vi "ODX_Ablaufbefehl.vi"(9 "Operand in":u32, 10 "Carry in":bool, 11 "SA2 Operator":T1[](array[typedef]) {"Wert" format="%.0x"}) -> (1 "Operand out":u32, 2 "Carry out":bool, 3 "SA2 Operator out":T1[](array[typedef]) {"Wert" format="%.0x"})   [LabVIEW 2014]
uses:
  Typedefs/Diagnose_SA2_Rechnenbefehl.ctl
  Typedefs/Diagnose_SA2_Operation_ENUM.ctl
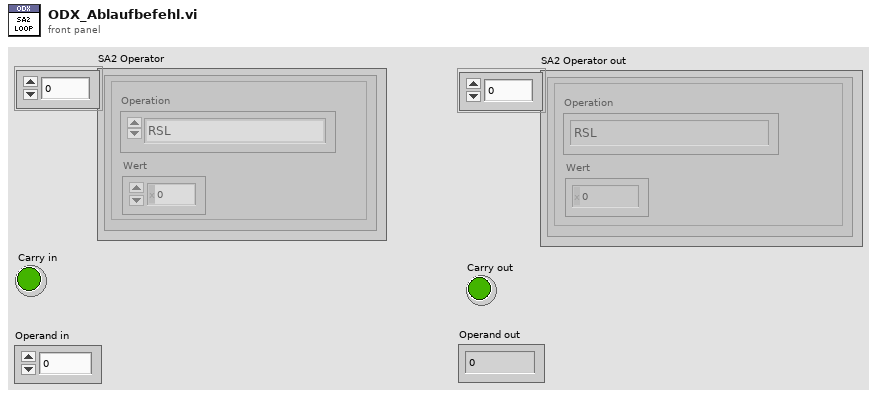
[diagram p1: front panel]
types:
  T1 = typedef "Diagnose_SA2_Rechnenbefehl.ctl" = cluster{"Operation":T2, "Wert":u32}
  T2 = typedef "Diagnose_SA2_Operation_ENUM.ctl" = enum16{"RSL", "RSR", "ADD", "SUB", "EOR", "Durchläufe", "NEXT", "BCC", "BRA", "Fertig"}
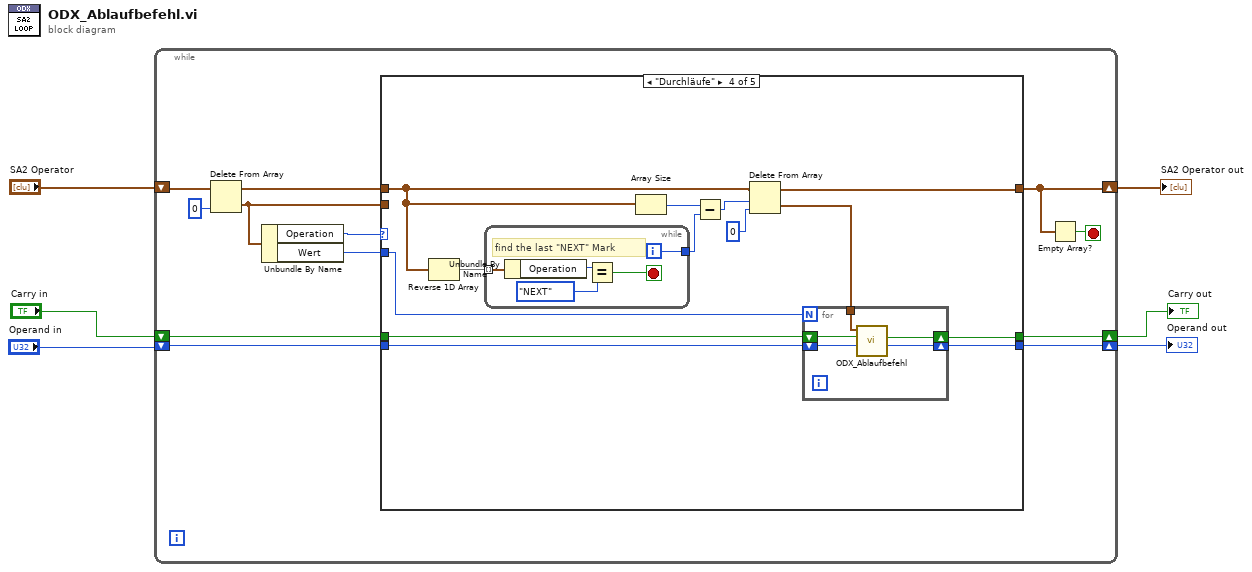
[diagram p0: block diagram]
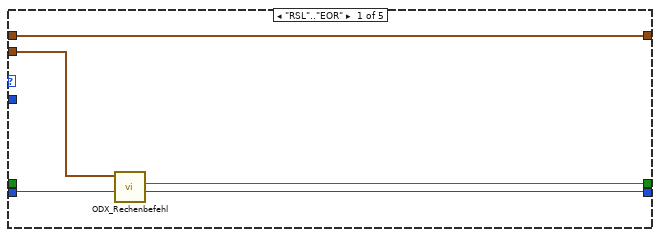
[diagram p2: hidden frame]
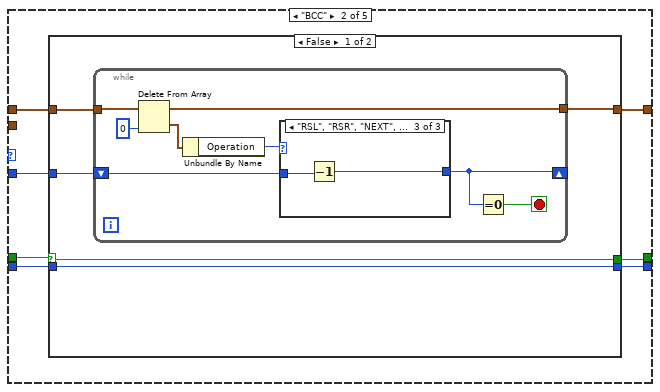
[diagram p3: hidden frame]
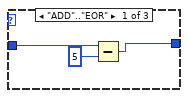
[diagram p4: hidden frame]
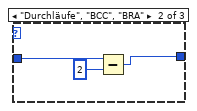
[diagram p5: hidden frame]
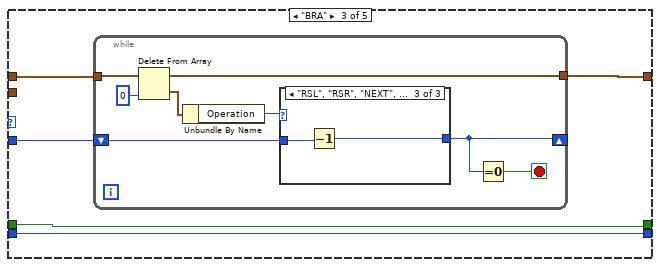
[diagram p7: hidden frame]
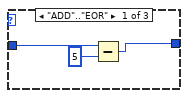
[diagram p8: hidden frame]
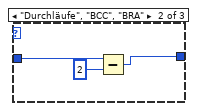
[diagram p9: hidden frame]
diagram:
  n1 = while {
    shift-right: [w16] -> w6
    shift-left: "Operand in" -> [w15]
    shift-right: [w7] -> w3
    shift-left: "SA2 Operator" -> [w14]
    shift-right: [w10] -> w1
    shift-left: "Carry in" -> [w9]
    stop <- w8 stop-if-true
    n2 = Delete From Array(array=w14, index=0) -> (deleted portion=w12:T1, array with subset deleted=w11:T1[])  [unwired: 1 in]
    n3 = Unbundle By Name(w12) -> ("Operation"=w18:T2, "Wert"=w17:u32)
    n4 = case shown="\"Durchläufe\"" w18 {
      tunnel: w17 -> [_ w24 w55 w76 _]
      tunnel: [w22 w28 w59 w79 w99] -> w16
      tunnel: w15 -> [w23 w29 w59 w80 w99]
      tunnel: w12 -> [w21 _ _ _ _]
      tunnel: w11 -> [w20 w27 w58 w85 w101]
      tunnel: [w20 w26 w57 w82 w101] -> w7
      tunnel: [w19 w25 w56 w78 w100] -> w10
      tunnel: w9 -> [_ w30 w56 w77 w100]
      frame "RSL".."EOR" {
        n5 = call "ODX_Rechenbefehl.vi"("Operand in"=w23, "operation"=w21) -> ("Operand out"=w22:u32, "Carry"=w19:bool)  [unwired: 8 in]
      }
      frame "BCC" {
        n6 = case shown="False" w30 {
          selector: w30 -> [w34 w52]
          tunnel: w29 -> [w35 w54]
          tunnel: [w35 w54] -> w28
          tunnel: [w31 w53] -> w26
          tunnel: w27 -> [w32 w53]
          tunnel: [w34 w52] -> w25
          tunnel: w24 -> [w33 _]
          frame False {
            n7 = while {
              shift-right: [w37] -> _
              shift-left: w33 -> [w38]
              tunnel: w32 -> [w43]
              tunnel: [w41] -> w31
              stop <- w36 stop-if-true
              n8 = Delete From Array(array=w43, index=0) -> (deleted portion=w40:T1, array with subset deleted=w41:T1[])  [unwired: 1 in]
              n9 = Unbundle By Name(w40) -> ("Operation"=w39:T2)
              n10 = case shown="\"RSL\", \"RSR\", \"NEXT\", \"Fertig\"" w39 {
                tunnel: w38 -> [w46 w49 w51]
                tunnel: [w44 w47 w50] -> w37
                frame "ADD".."EOR" {
                  n11 = Subtract(x=w46, y=u32 5) -> (x-y=w44:u32)
                }
                frame "Durchläufe", "BCC", "BRA" {
                  n12 = Subtract(x=w49, y=u32 2) -> (x-y=w47:u32)
                }
                frame "RSL", "RSR", "NEXT", "Fertig" {
                  n13 = Decrement(x=w51) -> (x-1=w50:u32)
                }
              }
              n14 = Equal To 0?(x=w37) -> (x = 0?=w36:bool)
            }
          }
          frame True {
          }
        }
      }
      frame "BRA" {
        n15 = while {
          shift-right: [w61] -> _
          shift-left: w55 -> [w62]
          tunnel: w58 -> [w67]
          tunnel: [w65] -> w57
          stop <- w60 stop-if-true
          n16 = Delete From Array(array=w67, index=0) -> (deleted portion=w64:T1, array with subset deleted=w65:T1[])  [unwired: 1 in]
          n17 = Unbundle By Name(w64) -> ("Operation"=w63:T2)
          n18 = case shown="\"RSL\", \"RSR\", \"NEXT\", \"Fertig\"" w63 {
            tunnel: w62 -> [w70 w73 w75]
            tunnel: [w68 w71 w74] -> w61
            frame "ADD".."EOR" {
              n19 = Subtract(x=w70, y=u32 5) -> (x-y=w68:u32)
            }
            frame "Durchläufe", "BCC", "BRA" {
              n20 = Subtract(x=w73, y=u32 2) -> (x-y=w71:u32)
            }
            frame "RSL", "RSR", "NEXT", "Fertig" {
              n21 = Decrement(x=w75) -> (x-1=w74:u32)
            }
          }
          n22 = Equal To 0?(x=w61) -> (x = 0?=w60:bool)
        }
      }
      frame "Durchläufe" {
        n23 = Reverse 1D Array(array=w85) -> (reversed array=w88:T1[])
        n24 = while {
          tunnel: w88 -> [w98] mode=indexing
          tunnel: [w94] -> w86
          i -> [w94]
          stop <- w95 stop-if-true
          # "find the last \"NEXT\" Mark"
          n25 = Unbundle By Name(w98) -> ("Operation"=w97:T2)
          n26 = Equal?(x=w97, y=Diagnose_SA2_Operation_ENUM."NEXT") -> (x = y?=w95:bool)
        }
        n27 = Array Size(array=w85) -> (size(s)=w87:i32)
        n28 = Subtract(x=w87, y=w86) -> (x-y=w84:i32)
        n29 = Delete From Array(array=w85, length=w84, index=0) -> (deleted portion=w81:T1[], array with subset deleted=w82:T1[])
        n30 = for {
          N: w76 -> [_]
          tunnel: w81 -> [w93]
          shift-right: [w91] -> w79
          shift-left: w80 -> [w92]
          shift-right: [w90] -> w78
          shift-left: w77 -> [w89]
          n31 = call "ODX_Ablaufbefehl.vi"("Operand in"=w92, "Carry in"=w89, "SA2 Operator"=w93) -> ("Operand out"=w91:u32, "Carry out"=w90:bool)  [unwired: 6 in, 1 out]
        }
      }
      frame "NEXT", "Fertig" {
      }
    }
    n32 = Empty Array?(array=w7) -> (empty?=w8:bool)
  }
  "Operand out" <- w6
  "SA2 Operator out" <- w3
  "Carry out" <- w1
